vi "2nd head.vi"(7 "second result":string, 8 "SN":string, 9 "midVar_time":string[](array[string]), 10 "second item name":string, 11 "second number":string) -> (3 "midVar_Content":string)   [LabVIEW 2011]
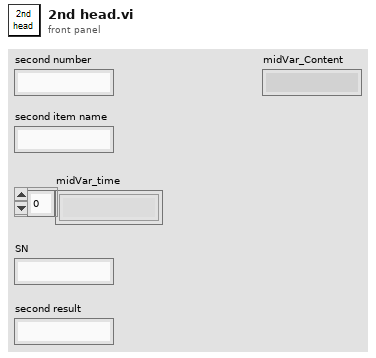
[diagram p1: front panel]
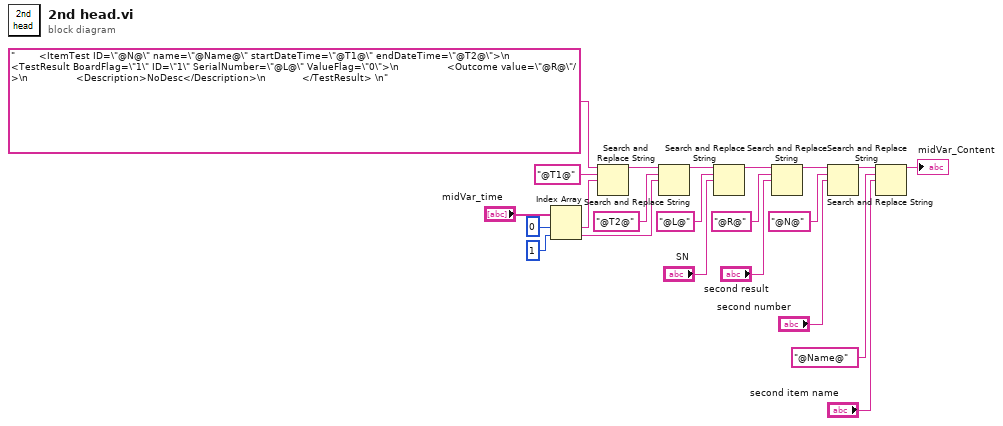
[diagram p0: block diagram]
diagram:
  n1 = Index Array(array="midVar_time", index #1=0 ("索引"), index #2=1 ("索引")) -> (element #1=w20:string, element #2=w17:string)
  n2 = Search and Replace String(input string="        <ItemTest ID=\"@N@\" name=\"@Name@\" startDateTime=\"@T1@\" endDateTime=\"@T2@\">\n            <TestResult BoardFlag=\"1\" ID=\"1\" SerialNumber=\"@L@\" ValueFlag=\"0\">\n                <Outcome value=\"@R@\"/>\n                <Description>NoDesc</Description>\n            </TestResult> \n", search string="@T1@" ("搜索字符串"), replace string=w20) -> (result string=w19:string)  [unwired: 5 in, 3 out]
  n3 = Search and Replace String(input string=w19, search string="@T2@" ("搜索字符串"), replace string=w17) -> (result string=w14:string)  [unwired: 5 in, 3 out]
  n4 = Search and Replace String(input string=w14, search string="@L@" ("搜索字符串"), replace string="SN") -> (result string=w12:string)  [unwired: 5 in, 3 out]
  n5 = Search and Replace String(input string=w12, search string="@R@" ("搜索字符串"), replace string="second result") -> (result string=w4:string)  [unwired: 5 in, 3 out]
  n6 = Search and Replace String(input string=w4, search string="@N@" ("搜索字符串"), replace string="second number") -> (result string=w3:string)  [unwired: 5 in, 3 out]
  n7 = Search and Replace String(input string=w3, search string="@Name@" ("搜索字符串"), replace string="second item name") -> (result string=→"midVar_Content":string)  [unwired: 5 in, 3 out]
